vi "dfd_Super Narrowband Filter Design CIC Filter Create Param.vi"(9 "ripple spec":T1={"passband"=0.1, "stopband"=40.0, "dB/linear? (T: dB)"=TRUE}, 10 "shaping original fstop":dbl, 11 "CIC factor":i32) -> (3 "CIC stage":i32)   [LabVIEW 2017, in "NI_DigFilter_Process.lvlib"]
uses:
  <vilib>/addons/Digital Filter Design/NI_DigFilter_Process.lvlib
  <vilib>/addons/Digital Filter Design/_Objects.llb/DFD Filter Ripple Specification (Design).ctl
  <vilib>/addons/Digital Filter Design/NI_DigFilter_Design.lvlib
  <vilib>/addons/Digital Filter Design/NI_DigFilterLicensed.lvlib
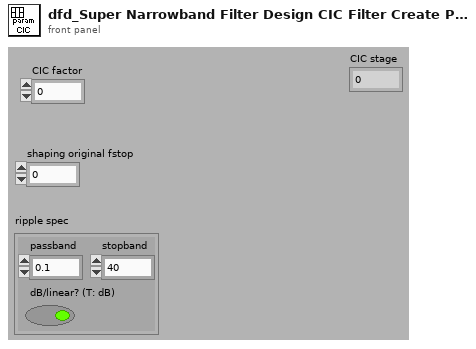
[diagram p1: front panel]
types:
  T1 = typedef "NI_DigFilterLicensed.lvlib/DFD Filter Ripple Specification (Design).ctl" = cluster{"passband":dbl, "stopband":dbl, "dB/linear? (T: dB)":bool}
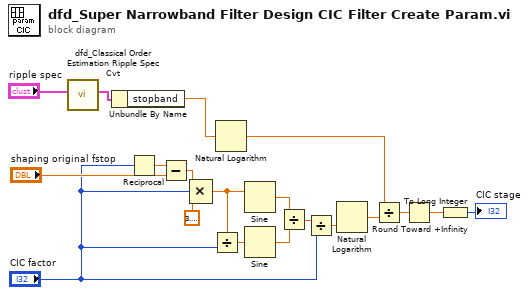
[diagram p0: block diagram]
diagram:
  n1 = call <vilib>:"dfd_Classical Order Estimation Ripple Spec Cvt.vi"("ripple specs"="ripple spec") -> ("ripple specs (linear)"=w1:T1)  [unwired: 10 out]
  n2 = Unbundle By Name(w1) -> ("stopband"=w2:dbl)
  n3 = Reciprocal(x="CIC factor") -> (1/x=w16:dbl)
  n4 = Subtract(x=w16, y="shaping original fstop") -> (x-y=w18:dbl)
  n5 = Compound Arithmetic op=MULTIPLY(w18, "CIC factor", 3.141592653589793) -> (w13:dbl)
  n6 = Divide(x=w13, y="CIC factor") -> (x/y=w7:dbl)
  n7 = Natural Logarithm(1:w2) -> (0:w11:dbl)
  n8 = Sine(x=w13) -> (sin(x)=w8:dbl)
  n9 = Sine(x=w7) -> (sin(x)=w9:dbl)
  n10 = Divide(x=w8, y=w9) -> (x/y=w10:dbl)
  n11 = Divide(x=w10, y="CIC factor") -> (x/y=w14:dbl)
  n12 = Natural Logarithm(1:w14) -> (0:w12:dbl)
  n13 = Divide(x=w11, y=w12) -> (x/y=w5:dbl)
  n14 = Round Toward +Infinity(x=w5) -> (ceil(x): smallest int >= x=w4:dbl)
  n15 = To Long Integer(number=w4) -> (32bit integer=→"CIC stage":i32)
